vi "TestSetOutWavePair.vi"(8 "error in (no error)":errorcluster) -> (0 "error out":errorcluster)   [LabVIEW 2019]
uses:
  <vilib>/addons/_JKI Toolkits/Caraya/classes/Test/Test.lvclass
  <vilib>/addons/_JKI Toolkits/Caraya/classes/Assert/Assert.lvclass
  <vilib>/addons/_JKI Toolkits/Caraya/classes/Assert/Assert Equal Value_Variant.vi
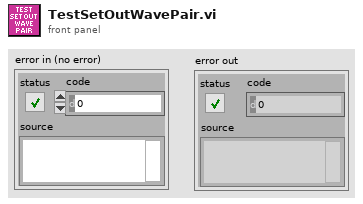
[diagram p1: front panel]
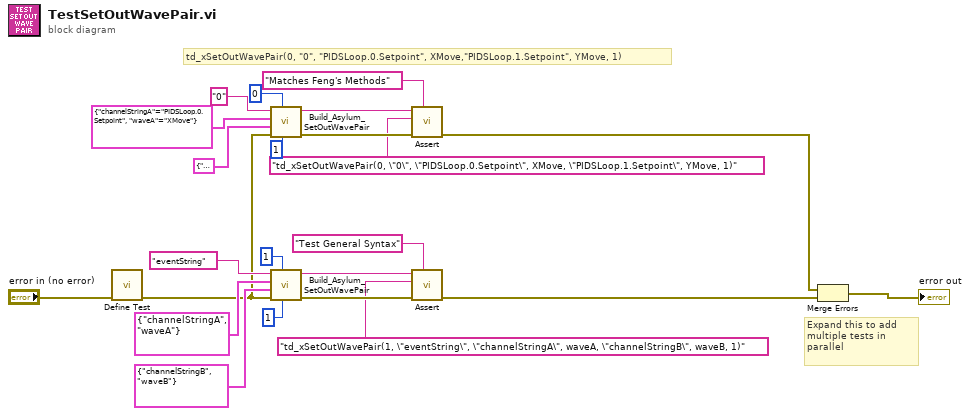
[diagram p0: block diagram]
diagram:
  # "td_xSetOutWavePair(0, \"0\", \"PIDSLoop.0.Setpoint\", XMove,\"PIDSLoop.1.Setpoint\", YMove, 1)"
  # "Expand this to add multiple tests in parallel"
  n1 = call <vilib>:"Define Test.vi"("error in (no error)"="error in (no error)") -> ("error out"=w6:errorcluster)  [unwired: 10 in]
  n2 = call "Build_Asylum_SetOutWavePair.vi"("interpolation"=1, "whichBank"=0, "error in (no error)"=w6, "Wave B"=cluster{"channelStringA":string, "waveA":string} {"channelStringA"="PIDSLoop.1.Setpoint", "waveA"="YMove"} ("Wave A"), "Wave A"=cluster{"channelStringA":string, "waveA":string} {"channelStringA"="PIDSLoop.0.Setpoint", "waveA"="XMove"}, "eventString"="0") -> ("error out"=w12:errorcluster, "Command"=w11:string)  [unwired: 4 in]
  n3 = call "Build_Asylum_SetOutWavePair.vi"("interpolation"=1, "whichBank"=1, "error in (no error)"=w6, "Wave B"=cluster{"channelString":string, "wave":string} {"channelString"="channelStringB", "wave"="waveB"} ("Wave"), "Wave A"=cluster{"channelString":string, "wave":string} {"channelString"="channelStringA", "wave"="waveA"} ("Wave"), "eventString"="eventString") -> ("error out"=w19:errorcluster, "Command"=w18:string)  [unwired: 4 in]
  n4 = call-poly <vilib>:"Assert.vi"("Label"="Matches Feng's Methods", "error in (no error)"=w12, "Y"="td_xSetOutWavePair(0, \"0\", \"PIDSLoop.0.Setpoint\", XMove, \"PIDSLoop.1.Setpoint\", YMove, 1)", "X"=w11) -> ("error out"=w3:errorcluster)  [unwired: 7 in]
  n5 = call-poly <vilib>:"Assert.vi"("Label"="Test General Syntax", "error in (no error)"=w19, "Y"="td_xSetOutWavePair(1, \"eventString\", \"channelStringA\", waveA, \"channelStringB\", waveB, 1)", "X"=w18) -> ("error out"=w21:errorcluster)  [unwired: 7 in]
  n6 = Merge Errors(w3, w21) -> (→"error out":errorcluster)
